vi "MARS_Read_TDMS_Properties.vi"(6 "Active Meas.":i32, 9 "Listbox":i32[](array[numeric])) -> ()   [LabVIEW 2015]
uses:
  ESA_Data_Analysis_Global_VIs.vi
  MARS_Global_var.vi
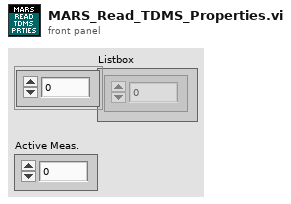
[diagram p1: front panel]
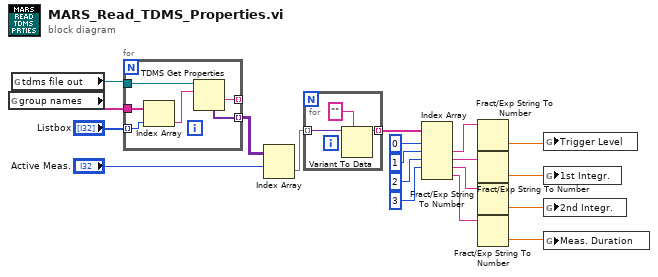
[diagram p0: block diagram]
diagram:
  n1 = global read "ESA_Data_Analysis_Global_VIs.vi" "group names"() -> (w5:string[])
  n2 = global read "ESA_Data_Analysis_Global_VIs.vi" "tdms file out"() -> (w6:refnum<k34>)
  n3 = for {
    tunnel: w6 -> [w25]
    tunnel: "Listbox" -> [w23] mode=indexing
    tunnel: w5 -> [w24]
    tunnel: [w21] -> w8 mode=indexing
    tunnel: [w20] -> _ mode=indexing
    n4 = Index Array(array=w24, index=w23) -> (element=w22:string)
    n5 = TDMS Get Properties(10:w22, 11:w25) -> (1:w20:string, 4:w21:variant[])  [unwired: 4 in, 4 out]
  }
  n6 = Index Array(array=w8, index (row)="Active Meas.") -> (element=w9:variant[])  [unwired: 1 in]
  n7 = for {
    tunnel: w9 -> [w27] mode=indexing
    tunnel: [w26] -> w11 mode=indexing
    n8 = Variant To Data(type="", Variant=w27) -> (data=w26:string)  [unwired: 1 in, 1 out]
  }
  n9 = Index Array(array=w11, index #1=0 ("index"), index #2=1 ("index"), index #3=2 ("index"), index #4=3 ("index")) -> (element #2=w16:string, element #3=w17:string, element #4=w18:string, element #5=w19:string)  [unwired: 1 in, 1 out]
  n10 = Fract/Exp String To Number(string=w16) -> (number=w4:dbl)  [unwired: 3 in, 1 out]
  n11 = Fract/Exp String To Number(string=w17) -> (number=w3:dbl)  [unwired: 3 in, 1 out]
  n12 = Fract/Exp String To Number(string=w18) -> (number=w2:dbl)  [unwired: 3 in, 1 out]
  n13 = Fract/Exp String To Number(string=w19) -> (number=w1:dbl)  [unwired: 3 in, 1 out]
  n14 = global write "MARS_Global_var.vi" "Trigger Level"(w4) -> ()
  n15 = global write "MARS_Global_var.vi" "1st Integr."(w3) -> ()
  n16 = global write "MARS_Global_var.vi" "2nd Integr."(w2) -> ()
  n17 = global write "MARS_Global_var.vi" "Meas. Duration"(w1) -> ()
